vi "Temperature Warnings.vi"(8 "에러 입력":cluster{"상태":bool, "코드":i32, "소스":string}, 11 "기상 데이터 입력":T1={"현재 온도"=0.0, "최고 온도"=0.0, "최저 온도"=0.0, "온도 경고?"=FALSE, "온도 경고 텍스트"="경고 없음"}) -> (0 "에러 출력":cluster{"상태":bool, "코드":i32, "소스":string}, 3 "기상 데이터 출력":T1={"현재 온도"=0.0, "최고 온도"=0.0, "최저 온도"=0.0, "온도 경고?"=FALSE, "온도 경고 텍스트"="경고 없음"})   [LabVIEW 2014]
doc: "이 VI는 현재 온도 및 리미트 설정에 기반하여 발행할 온도 경고의 정보를 결정하기 위해 사용됩니다."
uses:
  Weather Data.ctl
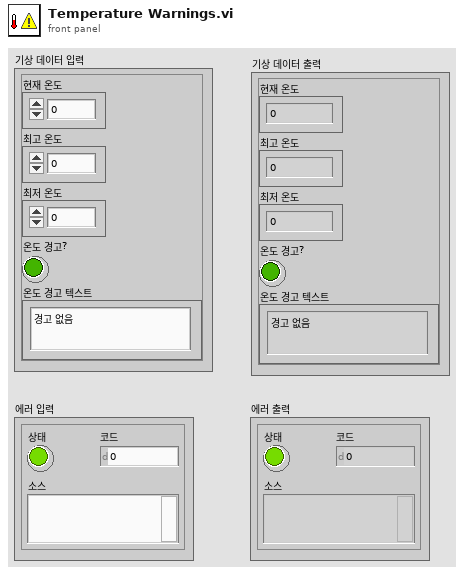
[diagram p1: front panel]
types:
  T1 = typedef "Weather Data.ctl" = cluster{"현재 온도":dbl, "최고 온도":dbl, "최저 온도":dbl, "온도 경고?":bool, "온도 경고 텍스트":string}
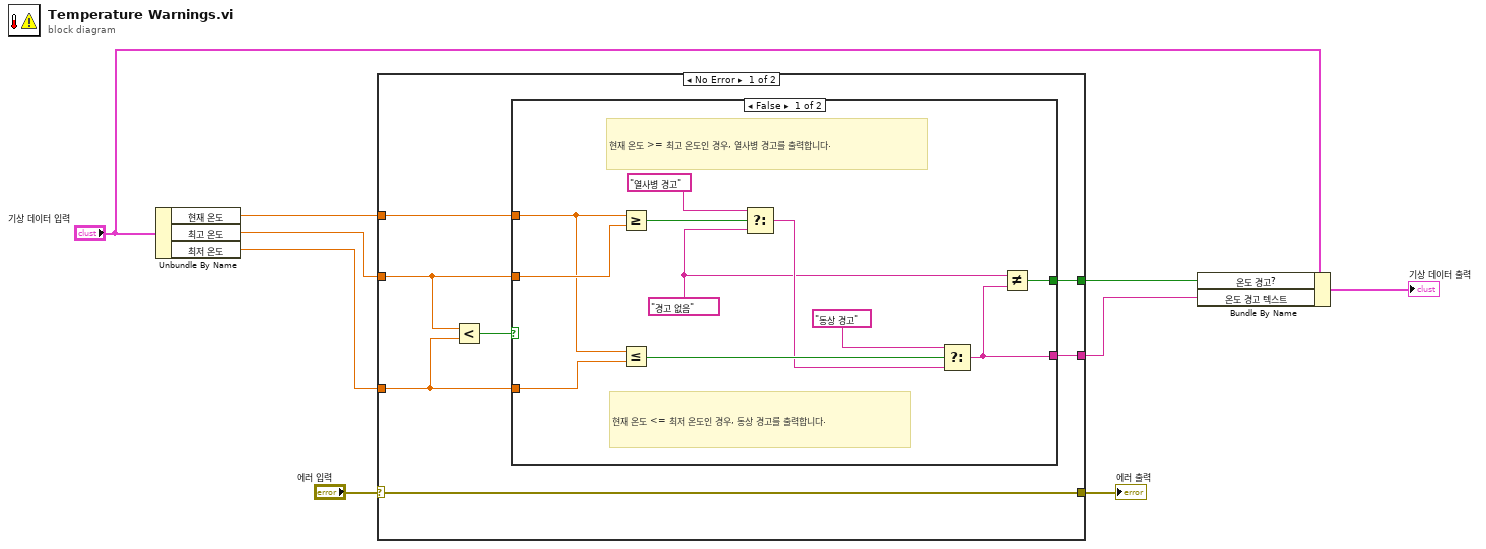
[diagram p0: block diagram]
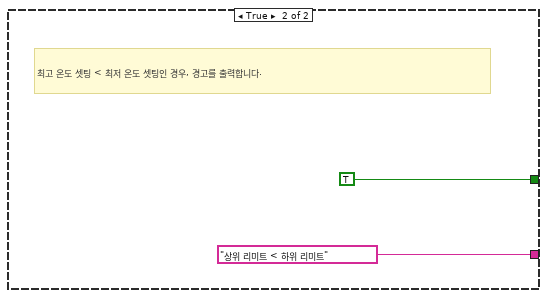
[diagram p2: hidden frame]
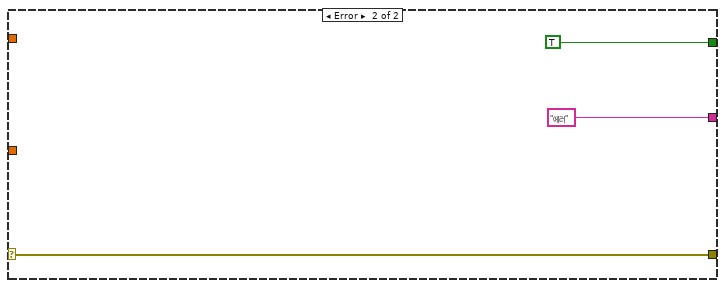
[diagram p3: hidden frame]
diagram:
  n1 = Unbundle By Name("기상 데이터 입력") -> ("현재 온도"=w7:dbl, "최고 온도"=w6:dbl, "최저 온도"=w5:dbl)
  n2 = case shown="No Error" "에러 입력" {
    selector: "에러 입력" -> [w14 w32]
    tunnel: [w16 "에러" ("f")] -> w4
    tunnel: [w15 TRUE] -> w3
    tunnel: [w14 w32] -> w8
    tunnel: w5 -> [w11 _]
    tunnel: w7 -> [w13 _]
    tunnel: w6 -> [w12 _]
    frame No Error {
      n3 = Less?(x=w12, y=w11) -> (x < y?=w10:bool)
      n4 = case shown="False" w10 {
        tunnel: [w17 "상위 리미트 < 하위 리미트" ("f")] -> w16
        tunnel: [w27 TRUE] -> w15
        tunnel: w12 -> [w26 _]
        tunnel: w11 -> [w23 _]
        tunnel: w13 -> [w19 _]
        frame False {
          w18 = "경고 없음" ("f")
          # "현재 온도 <= 최저 온도인 경우, 동상 경고를 출력합니다."
          # "현재 온도 >= 최고 온도인 경우, 열사병 경고를 출력합니다."
          n5 = Greater Or Equal?(x=w19, y=w26) -> (x >= y?=w25:bool)
          n6 = Less Or Equal?(x=w19, y=w23) -> (x <= y?=w21:bool)
          n7 = Select(t="열사병 경고", s=w25, f=w18) -> (s? t:f=w20:string)
          n8 = Select(t="동상 경고", s=w21, f=w20) -> (s? t:f=w17:string)
          n9 = Not Equal?(x=w18, y=w17) -> (x != y?=w27:bool)
        }
        frame True {
          # "최고 온도 셋팅 < 최저 온도 셋팅인 경우, 경고를 출력합니다."
        }
      }
    }
    frame Error {
    }
  }
  "에러 출력" <- w8
  n10 = Bundle By Name(cluster="기상 데이터 입력", "온도 경고?"=w3, "온도 경고 텍스트"=w4) -> (→"기상 데이터 출력":T1)
